vi "RIO_CheckPrecidence.vi"(2 "new op":string, 3 "last op":string) -> (0 "lower precidence?":bool, 1 "transidental end?":bool)   [LabVIEW 2012]
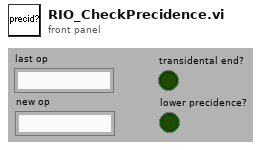
[diagram p1: front panel]
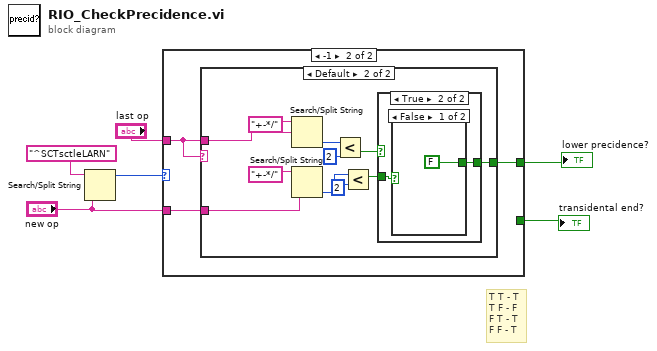
[diagram p0: block diagram]
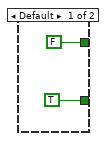
[diagram p2: hidden frame]
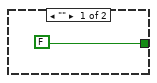
[diagram p3: hidden frame]
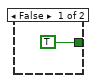
[diagram p4: hidden frame]
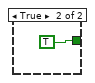
[diagram p5: hidden frame]
diagram:
  # "T T - T\nT F - F\nF T - T\nF F - T"
  n1 = Search/Split String(string="^SCTsctleLARN" ("String"), search string/char (-)="new op") -> (offset of match=w2:i32)  [unwired: 1 in, 2 out]
  n2 = case shown="-1" w2 {
    tunnel: [FALSE w11] -> w6
    tunnel: "last op" -> [_ w10]
    tunnel: "new op" -> [_ w9]
    tunnel: [TRUE _] -> w1
    frame Default {
    }
    frame -1 {
      n3 = case shown="Default" w10 {
        tunnel: w10 -> [_ w22]
        tunnel: [FALSE w14] -> w11
        tunnel: w9 -> [_ w13]
        frame "" {
        }
        frame Default {
          n4 = Search/Split String(string="+-*/" ("String"), search string/char (-)=w22) -> (offset of match=w18:i32)  [unwired: 1 in, 2 out]
          n5 = Search/Split String(string="+-*/" ("String"), search string/char (-)=w13) -> (offset of match=w19:i32)  [unwired: 1 in, 2 out]
          n6 = Less?(x=w18, y=2) -> (x < y?=w16:bool)
          n7 = Less?(x=w19, y=2) -> (x < y?=w15:bool)
          n8 = case shown="True" w16 {
            tunnel: w15 -> [_ w26]
            tunnel: [TRUE w25] -> w14
            frame False {
            }
            frame True {
              n9 = case shown="False" w26 {
                tunnel: [FALSE TRUE] -> w25
                frame False {
                }
                frame True {
                }
              }
            }
          }
        }
      }
    }
  }
  "lower precidence?" <- w6
  "transidental end?" <- w1
